vi "Terminate Data Notifications.vi"(8 "error in (no error)":errorcluster, 11 "Task Base in":refnum<class "Task Base.lvclass">) -> (0 "error out":errorcluster, 3 "Task Base out":refnum<class "Task Base.lvclass">)   [LabVIEW 2023, in "HAL GOOP4.lvlib" / "Task Base.lvclass"]
uses:
  Task Base.lvclass
  Task Base.lvclass/Task Base.ctl
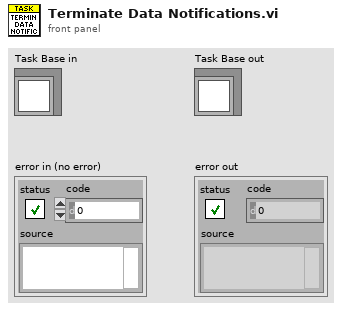
[diagram p1: front panel]
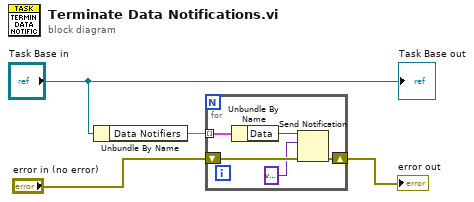
[diagram p0: block diagram]
diagram:
  n1 = Unbundle By Name("Task Base in") -> ("Data Notifiers"=w3:map{string, refnum<notifier>})
  n2 = for {
    tunnel: w3 -> [w9] mode=indexing
    shift-right: [w7] -> w1
    shift-left: "error in (no error)" -> [w8]
    n3 = Unbundle By Name(w9) -> ("Data"=w5:refnum<notifier>)
    n4 = Send Notification(notification=variant, notifier=w5, error in (no error)=w8) -> (error out=w7:errorcluster)  [unwired: 1 out]
  }
  "error out" <- w1
  "Task Base out" <- "Task Base in"
